vi "truthTableSubVI.vi"(0 "Numeric":dbl) -> (1 "Boolean":bool=TRUE, 2 "Boolean 2":bool=TRUE, 3 "Boolean 3":bool=TRUE, 4 "Boolean 4":bool=TRUE)   [LabVIEW 2015]
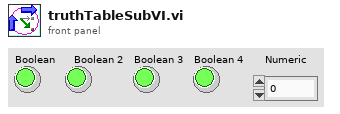
[diagram p1: front panel]
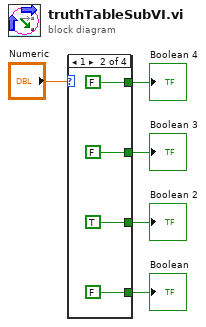
[diagram p0: block diagram]
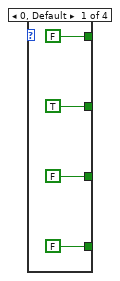
[diagram p2: hidden frame]
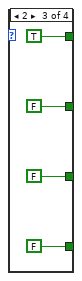
[diagram p3: hidden frame]
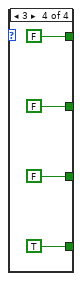
[diagram p4: hidden frame]
diagram:
  n1 = case shown="1" "Numeric" {
    tunnel: [FALSE FALSE FALSE TRUE] -> w4
    tunnel: [FALSE TRUE FALSE FALSE] -> w3
    tunnel: [TRUE FALSE FALSE FALSE] -> w2
    tunnel: [FALSE FALSE TRUE FALSE] -> w1
    frame 0, Default {
    }
    frame 1 {
    }
    frame 2 {
    }
    frame 3 {
    }
  }
  "Boolean" <- w4
  "Boolean 2" <- w3
  "Boolean 3" <- w2
  "Boolean 4" <- w1
